vi "Read Global Locked.vi"(7 "Semaphore Timeout":i32=-1, 8 "error in (no error)":errorcluster, 11 "DriveMotorsLeft in":refnum<class "DriveMotorsLeft.lvclass">) -> (0 "error out":errorcluster, 1 "Semaphore Timed Out":bool, 2 "Global":refnum<class "System.lvclass">, 3 "DriveMotorsLeft out":refnum<class "DriveMotorsLeft.lvclass">)   [LabVIEW 2013]
uses:
  Robot Global Data.vi
  System/System.lvclass
  DriveMotorsLeft.lvclass
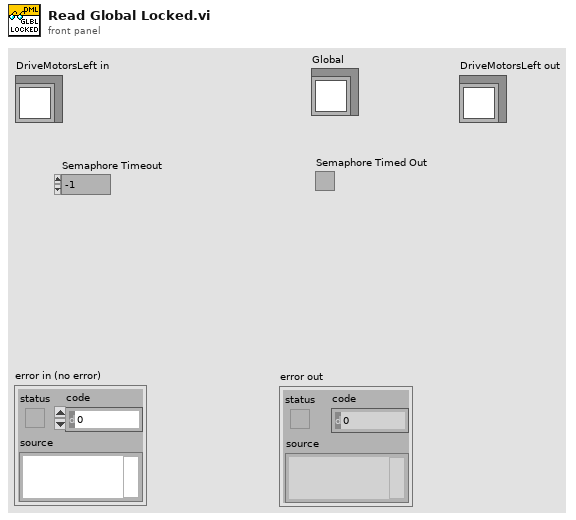
[diagram p1: front panel]
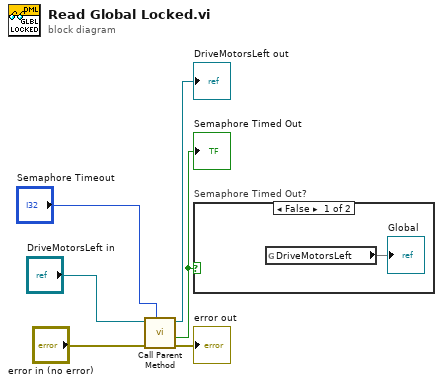
[diagram p0: block diagram]
diagram:
  n1 = call-parent "Call Parent Method"("Semaphore Timeout"="Semaphore Timeout", "error in (no error)"="error in (no error)", "System in"="DriveMotorsLeft in") -> ("error out"=→"error out":errorcluster, "Semaphore Timed Out"=w2:bool, "System out"=→"DriveMotorsLeft out":refnum<class "DriveMotorsLeft.lvclass">)  [unwired: 5 in, 1 out]
  "Semaphore Timed Out" <- w2
  n2 = case "Semaphore Timed Out?" shown="False" w2 {
    frame False {
      n3 = global read "Robot Global Data.vi" "DriveMotorsLeft"() -> (→"Global")
    }
    frame True {
    }
  }
